vi "BusTapeFiducialAnalysis.vi"() -> ()   [LabVIEW 2016]
uses:
  <vilib>/vision/Image Controls.llb/IMAQ Image.ctl
  <vilib>/vision/Measure.llb/Edge Options.ctl
  <vilib>/vision/Measure.llb/Edge Polarity.ctl
  <vilib>/Analysis/6fits.llb/Curve Fitting Criteria.ctl
  <vilib>/Utility/file.llb/Write Delimited Spreadsheet (DBL).vi
  <vilib>/vision/NI_Vision_Development_Module.lvlib
  <vilib>/Analysis/NI_AALPro.lvlib
  <vilib>/Analysis/NI_AALBase.lvlib
panel:
  out "Std Dev":dbl
  out "Mean":dbl
  out "Fit Deviation":T1(graph)
  out "Fiducial spacing (mm)\n(bottom)":dbl[](array[numeric])
  out "Fiducial spacing (mm)\n(top)":dbl[](array[numeric])
  out "Deviation from Fit (um)":dbl[](array[numeric])
  out "Mean Location Error (um)":dbl[][](array[numeric])
  out "Mean Location (mm)":dbl[][](array[numeric])
  out "Fiducial 14 Y":cluster{i32[], dbl[]}(graph)
  out "Fiducial 14 X":cluster{i32[], dbl[]}(graph)
  out "Fiducial 13 Y":cluster{i32[], dbl[]}(graph)
  out "Fiducial 13 X":cluster{i32[], dbl[]}(graph)
  out "Fiducial 12 Y":cluster{i32[], dbl[]}(graph)
  out "Fiducial 12 X":cluster{i32[], dbl[]}(graph)
  out "Fiducial 11 Y":cluster{i32[], dbl[]}(graph)
  out "Fiducial 11 X":cluster{i32[], dbl[]}(graph)
  out "Fiducial 10 Y":cluster{i32[], dbl[]}(graph)
  out "Fiducial 10 X":cluster{i32[], dbl[]}(graph)
  out "Fiducial 9 Y":cluster{i32[], dbl[]}(graph)
  out "Fiducial 9 X":cluster{i32[], dbl[]}(graph)
  out "Fiducial 8 Y":cluster{i32[], dbl[]}(graph)
  out "Fiducial 8 X":cluster{i32[], dbl[]}(graph)
  out "Fiducial 7 Y":cluster{i32[], dbl[]}(graph)
  out "Fiducial 7 X":cluster{i32[], dbl[]}(graph)
  out "Fiducial 6 Y":cluster{i32[], dbl[]}(graph)
  out "Fiducial 6 X":cluster{i32[], dbl[]}(graph)
  out "Fiducial 5 Y":cluster{i32[], dbl[]}(graph)
  out "Fiducial 5 X":cluster{i32[], dbl[]}(graph)
  out "Fiducial 4 Y":cluster{i32[], dbl[]}(graph)
  out "Fiducial 4 X":cluster{i32[], dbl[]}(graph)
  out "Fiducial 3 Y":cluster{i32[], dbl[]}(graph)
  out "Fiducial 3 X":cluster{i32[], dbl[]}(graph)
  out "Fiducial 2 Y":cluster{i32[], dbl[]}(graph)
  out "Fiducial 2 X":cluster{i32[], dbl[]}(graph)
  out "Fiducial 1 Y":cluster{i32[], dbl[]}(graph)
  out "Fiducial 1 X":cluster{i32[], dbl[]}(graph)
  out "Fiducial Loc":dbl[][](array[numeric])
  out "Drift 2":cluster{dbl[], dbl[]}(graph)
  out "Radius [um] 2":dbl[](array[numeric])
  out "Derivative: Normalized Intensity vs Radius":T2(graph)
  out "Normalized Intensity vs Radius":cluster{dbl[], dbl[]}(graph)
  in  "nBins":dbl=300.0
  in  "Min":dbl
  in  "Max":dbl=300.0
  out "Npixel@Intensity Histogram":T1(graph)
  out "Npixel@phi Histogram":T1(graph)
  out "Npixel@R Histogram":T1(graph)
  out "Bottom Intercept\n(mm)":dbl
  out "Bottom Slope\n(um/mm)":dbl
  out "Top Intercept\n(mm)":dbl
  out "Top Slope\n(um/mm)":dbl
  out "Pixel to Micron Conversion":T1(graph)
  out "Bottom errors (um)":dbl[](array[numeric])
  out "Top errors (um)":dbl[](array[numeric])
  out "Scaling [um/px]":dbl[](array[numeric])
  out "Bottom":cluster{"Bottom":dbl[], "Bottom":dbl[]}[](graph)
  out "Bottom \nResiduals (um)":dbl[](array[numeric])
  out "Radius [um]":dbl[](array[numeric])
  out "Top \nResiduals (um)":dbl[](array[numeric])
  out "Top":cluster{"Top":dbl[], "Top":dbl[]}[](graph)
  in  "method":T3 items=["Least Square", "Least Absolute Residual", "Bisquare"]
  out "Bottom":dbl[][](array[numeric])
  out "Top":dbl[][](array[numeric])
  out "Coordinate array for image capture":dbl[][](array[numeric])
  out "Processing Image #":i32
  out "Selected subarray":T4(plugin-control)
  out "Fitted Circle":T5 {"Average SNR (dB)" format="%.2f"; "Average Strength" format="%.2f"; "Roundness (Real-World)" format="%.2f"; "Radius (Real-World)" format="%.2f"; "Center (Real-World)"."Y" format="%.2f"; "Center (Real-World)"."X" format="%.2f"; "Radius (Pixels)" format="%.2f"; "Center (Pixels)"."Y" format="%.2f"; "Center (Pixels)"."X" format="%.2f"}
  in  "Circle ROI Descriptor":T6={"Global Rectangle"=[675, 567, 1751, 1642], "Contours"=[{"ID"=enum."External", "Type"=7, "Coordinates"=[1212, 1104, 190, 250, 0, 0]}]} {"Contours"."Type" items=["No Selection", "Point", "Line", "Rectangle", "Oval", "Polygon", "Freehand Region", "Annulus", "Unused2", "Unused3", "Broken Line", "Freehand Line", "Rotated Rectangle"]}
  in  "Circle Fit Options":T7={"Process"=enum."Get Best Edge", "Step Size"=3.0, "Max Pixel Radius"=3}
  in  "Circle Finding Options":T10={"Search  Direction"=1, "Edge Options"={"Edge Polarity"=2, "Kernel Size"=3, "Width"=3, "Minimum Edge Strength"=10.0, "Interpolation Type"=enum."Bilinear Fixed", "Data Processing Method"=enum."Median"}, "Show Search Area"=TRUE, "Show Search Lines"=TRUE, "Show Edges Found"=TRUE, "Show Result"=TRUE, "Search Area Color"=65280, "Search Lines Color"=255, "Edge Locations Color"=16776960, "Result Color"=65511, "Overlay Group Name"=""} {"Search  Direction" items=["Outside to Inside", "Inside to Outside"]; "Edge Options"."Edge Polarity" items=["All Edges", "Rising Edges", "Falling Edges"]; "Edge Options"."Minimum Edge Strength" format="%.2f"; "Edge Options"."Width" step=2; "Edge Options"."Kernel Size" step=2}
  in  "Pattern Match Settings":T11={"Algorithm"=2, "Number of Matches Requested"=1, "Minimum Match Score"=800.0, "SubPixel Accuracy"=TRUE, "Rotation Angle Ranges"=[], "Show Search Area"=FALSE, "Show Result"=TRUE} {"Rotation Angle Ranges"."End" format="%.1f"; "Rotation Angle Ranges"."Start" format="%.1f"; "Minimum Match Score" min=0 max=1000 format="%.2f"; "Number of Matches Requested" min=1; "Algorithm" items=["All", "Low Discrepancy Sampling", "Grayscale Value Pyramid", "Gradients Pyramid"]}
  out "Template Image":T4
  in  "Coordinate file for image capture":path=path "D:/Git/StaveAssembly/XYZstage+Camera_CollectedImages/2017-03-15/BrendonsFidMarks_dots_2017-03-15-captured.csv"
  out "Review":bool
  out "Search running?":bool
  in  "Stop and delete":bool
  out "Images Array":T4[](array[plugin-control])=["image_442_-22_00"]
  in  "error in":errorcluster
  out "error out":errorcluster
  out "Filenames Array":string[](array[string])=["image_442_-22_110.png", "image_442_-22_137.png", "image_442_-22_192.png", "image_442_-22_222.png", "image_442_-22_26.png", "image_442_-22_56.png"]
  in  "Naming Convention":string="image_*_*_*_*.png"
  in  "Images Directory":path=path "D:/Git/StaveAssembly/XYZstage+Camera_CollectedImages/2017-03-15/images"
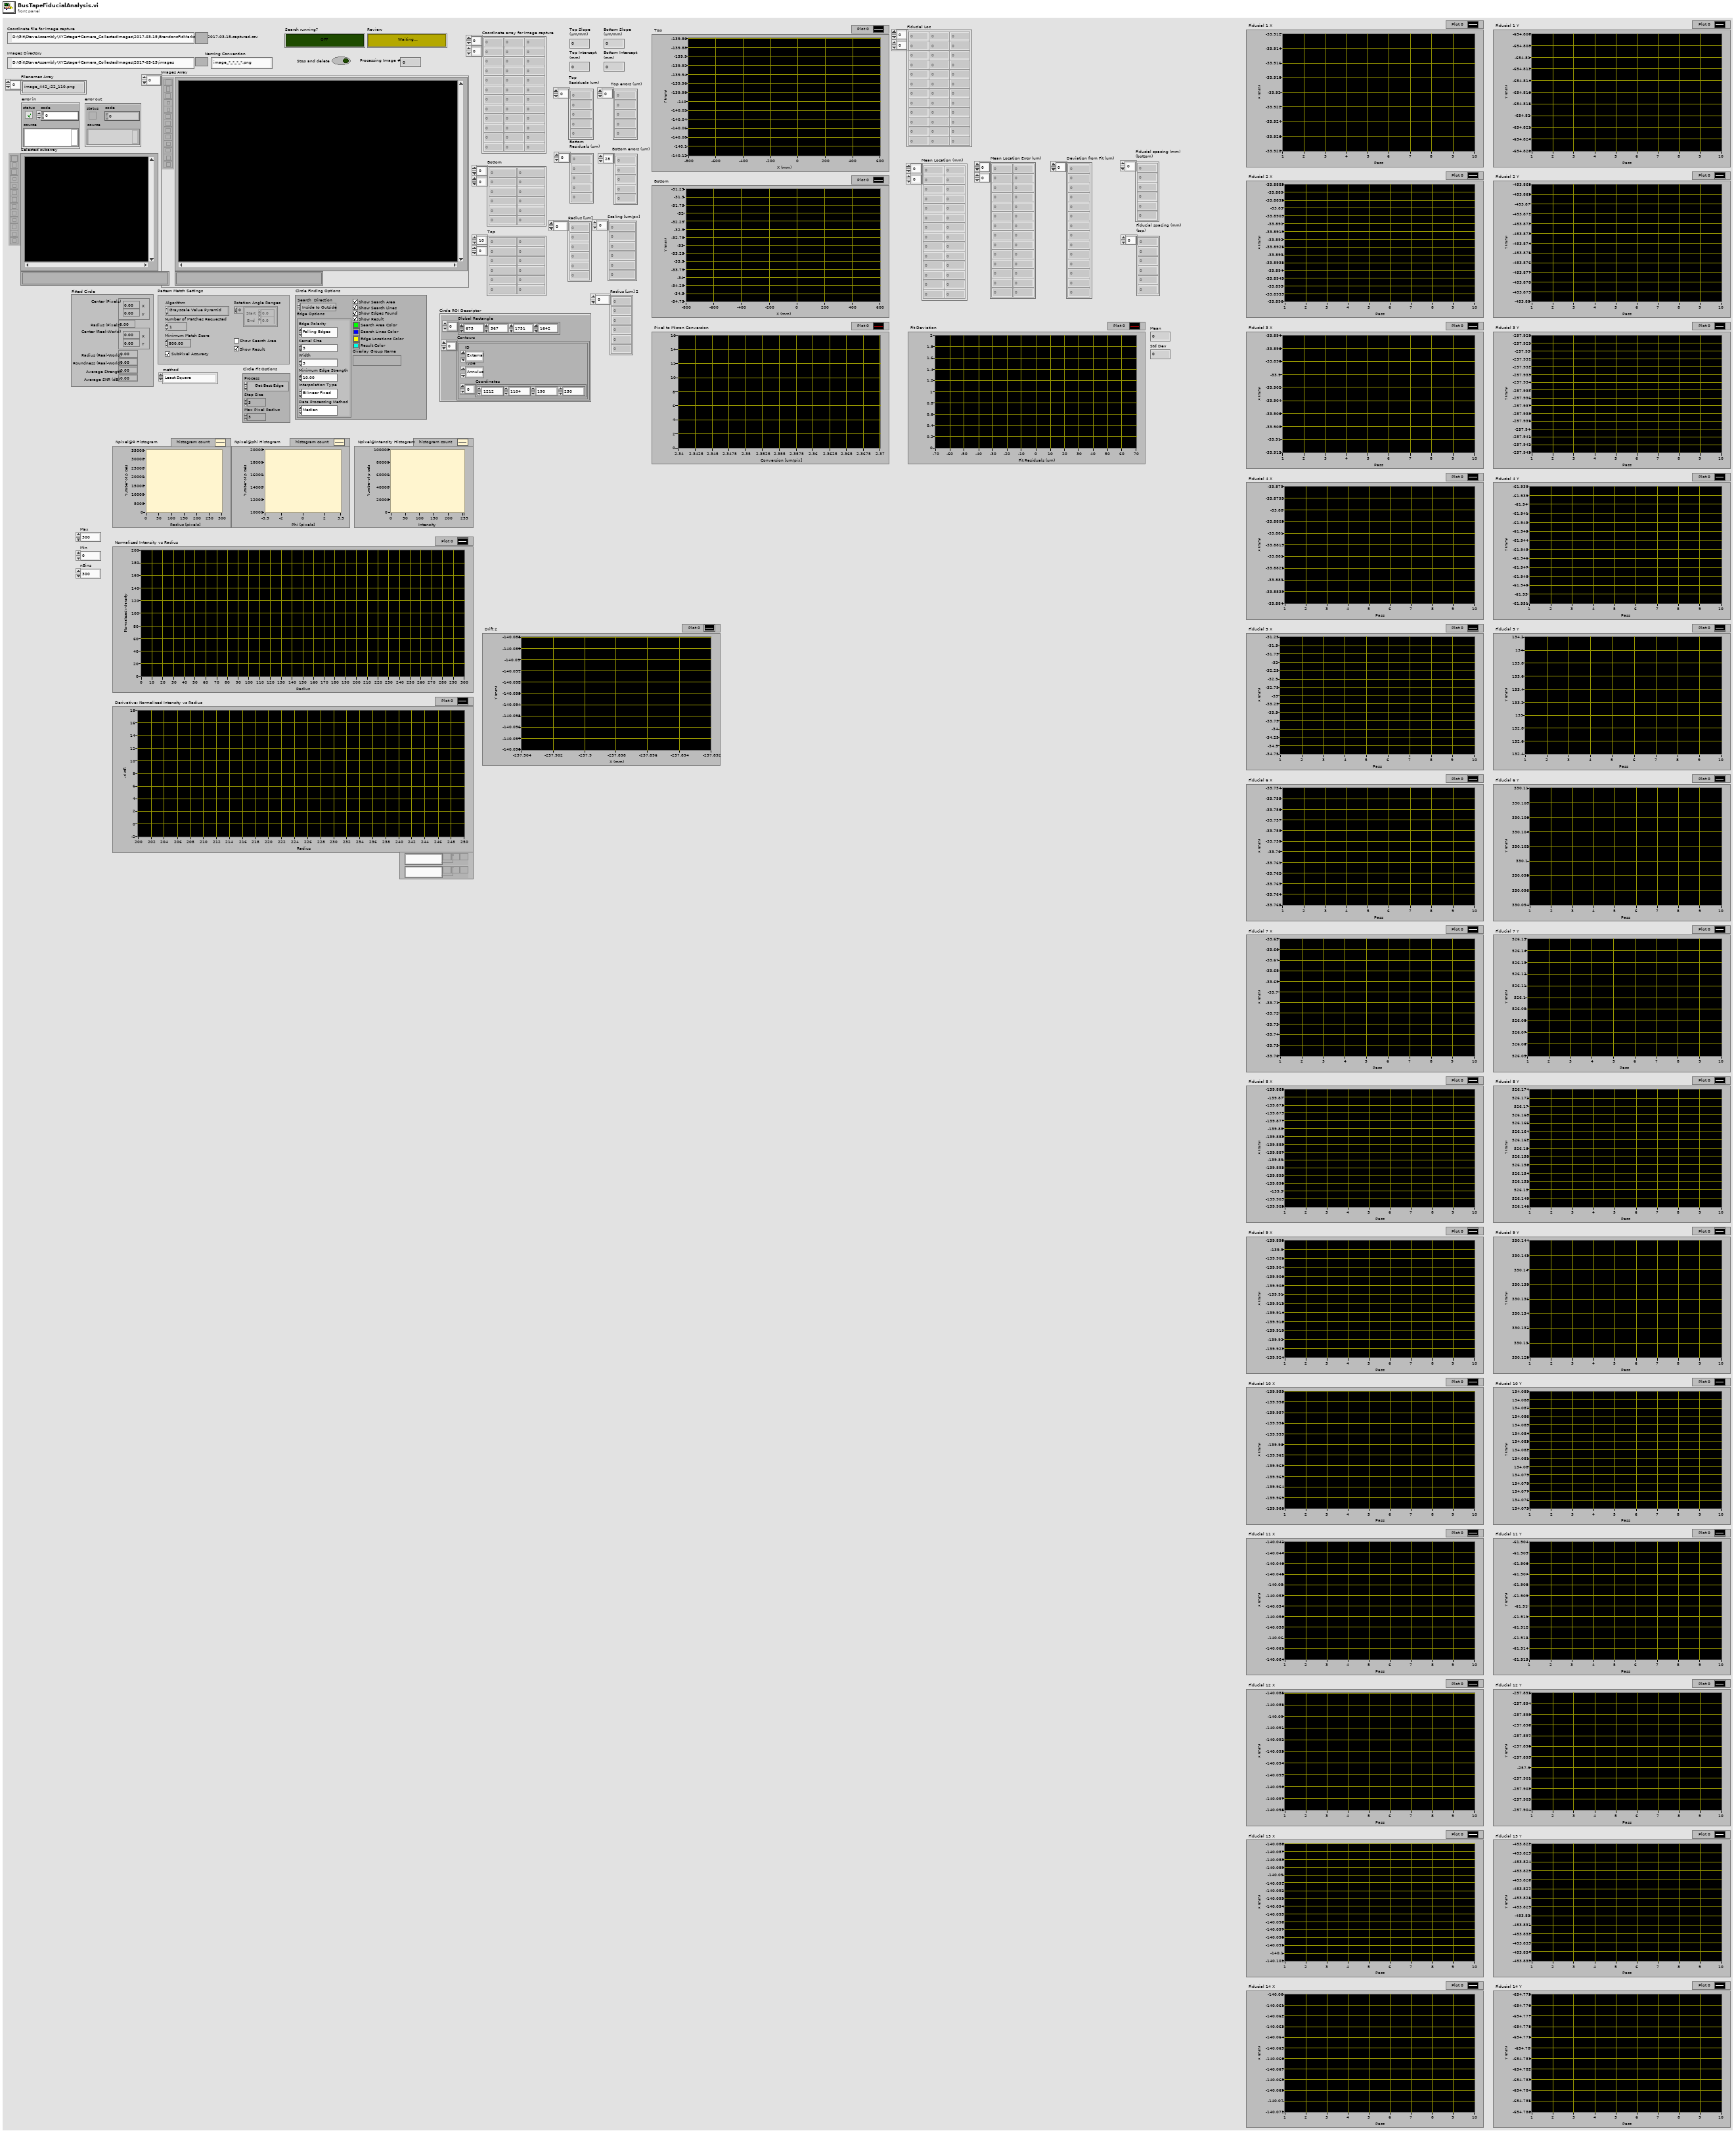
[diagram p1: front panel]
types:
  T1 = cluster{"X Values":dbl[], "Histogram: h(x)":i32[]}
  T2 = cluster{"Radius bins":dbl[], "Best Gaussian Fit":dbl[]}[]
  T3 = typedef "NI_AALPro.lvlib/Curve Fitting Criteria.ctl" = u16
  T4 = typedef "IMAQ Image.ctl" = refnum<image>
  T5 = cluster{"Center (Pixels)":cluster{"X":sgl, "Y":sgl}, "Radius (Pixels)":dbl, "Center (Real-World)":cluster{"X":sgl, "Y":sgl}, "Radius (Real-World)":dbl, "Roundness (Real-World)":dbl, "Average Strength":dbl, "Average SNR (dB)":dbl}
  T6 = cluster{"Global Rectangle":i32[], "Contours":cluster{"ID":enum32{"External", "Internal"}, "Type":u32, "Coordinates":i32[]}[]}
  T7 = cluster{"Process":enum16{"Get First Edge", "Get First + Last Edge", "Get All Edges", "Get Best Edge"}, "Step Size":dbl, "Max Pixel Radius":i32}
  T8 = typedef "Edge Options.ctl" = cluster{"Edge Polarity":T9, "Kernel Size":u32, "Width":u32, "Minimum Edge Strength":sgl, "Interpolation Type":enum32{"Zero Order", "Bilinear", "Quadratic", "Cubic", "Bilinear Fixed"}, "Data Processing Method":enum32{"Average", "Median"}}
  T9 = typedef "Edge Polarity.ctl" = u32
  T10 = cluster{"Search  Direction":u32, "Edge Options":T8, "Show Search Area":bool, "Show Search Lines":bool, "Show Edges Found":bool, "Show Result":bool, "Search Area Color":u32, "Search Lines Color":u32, "Edge Locations Color":u32, "Result Color":u32, "Overlay Group Name":string}
  T11 = cluster{"Algorithm":i32, "Number of Matches Requested":i32, "Minimum Match Score":sgl, "SubPixel Accuracy":bool, "Rotation Angle Ranges":cluster{"Start":sgl, "End":sgl}[], "Show Search Area":bool, "Show Result":bool}
  T12 = enum16{"Get First Edge", "Get First + Last Edge", "Get All Edges", "Get Best Edge"}
  T13 = typedef "Search Line.ctl" = cluster{"Start Point":cluster{"X":sgl, "Y":sgl}, "End Point":cluster{"X":sgl, "Y":sgl}, "Edge Info":T14[], "Edge Map":dbl[], "Calibration Valid":bool}
  T14 = typedef "Edge New.ctl" = cluster{"Location (Pixel)":cluster{"X":sgl, "Y":sgl}, "Location (Real-World)":cluster{"X":sgl, "Y":sgl}, "Distance (Pixel)":dbl, "Distance (Real-World)":dbl, "Strength":dbl, "Noise":dbl, "Rising?":bool}
  T15 = cluster{"Position":cluster{"x":sgl, "y":sgl}, "Angle":sgl, "Scale":sgl, "Score":sgl, "Bounding Box":cluster{"x":sgl, "y":sgl}[]}[]
  T16 = cluster{"Global Rectangle":i32[], cluster{"ID":enum32{"External", "Internal"}, "Type":u32, "Coordinates":i32[]}[]}
  T17 = cluster{"initial amplitude":dbl, "initial center":dbl, "initial standard deviation":dbl, "offset":dbl}
  T18 = cluster{"Radius bins":dbl[], "Normalized Intensity":dbl[]}
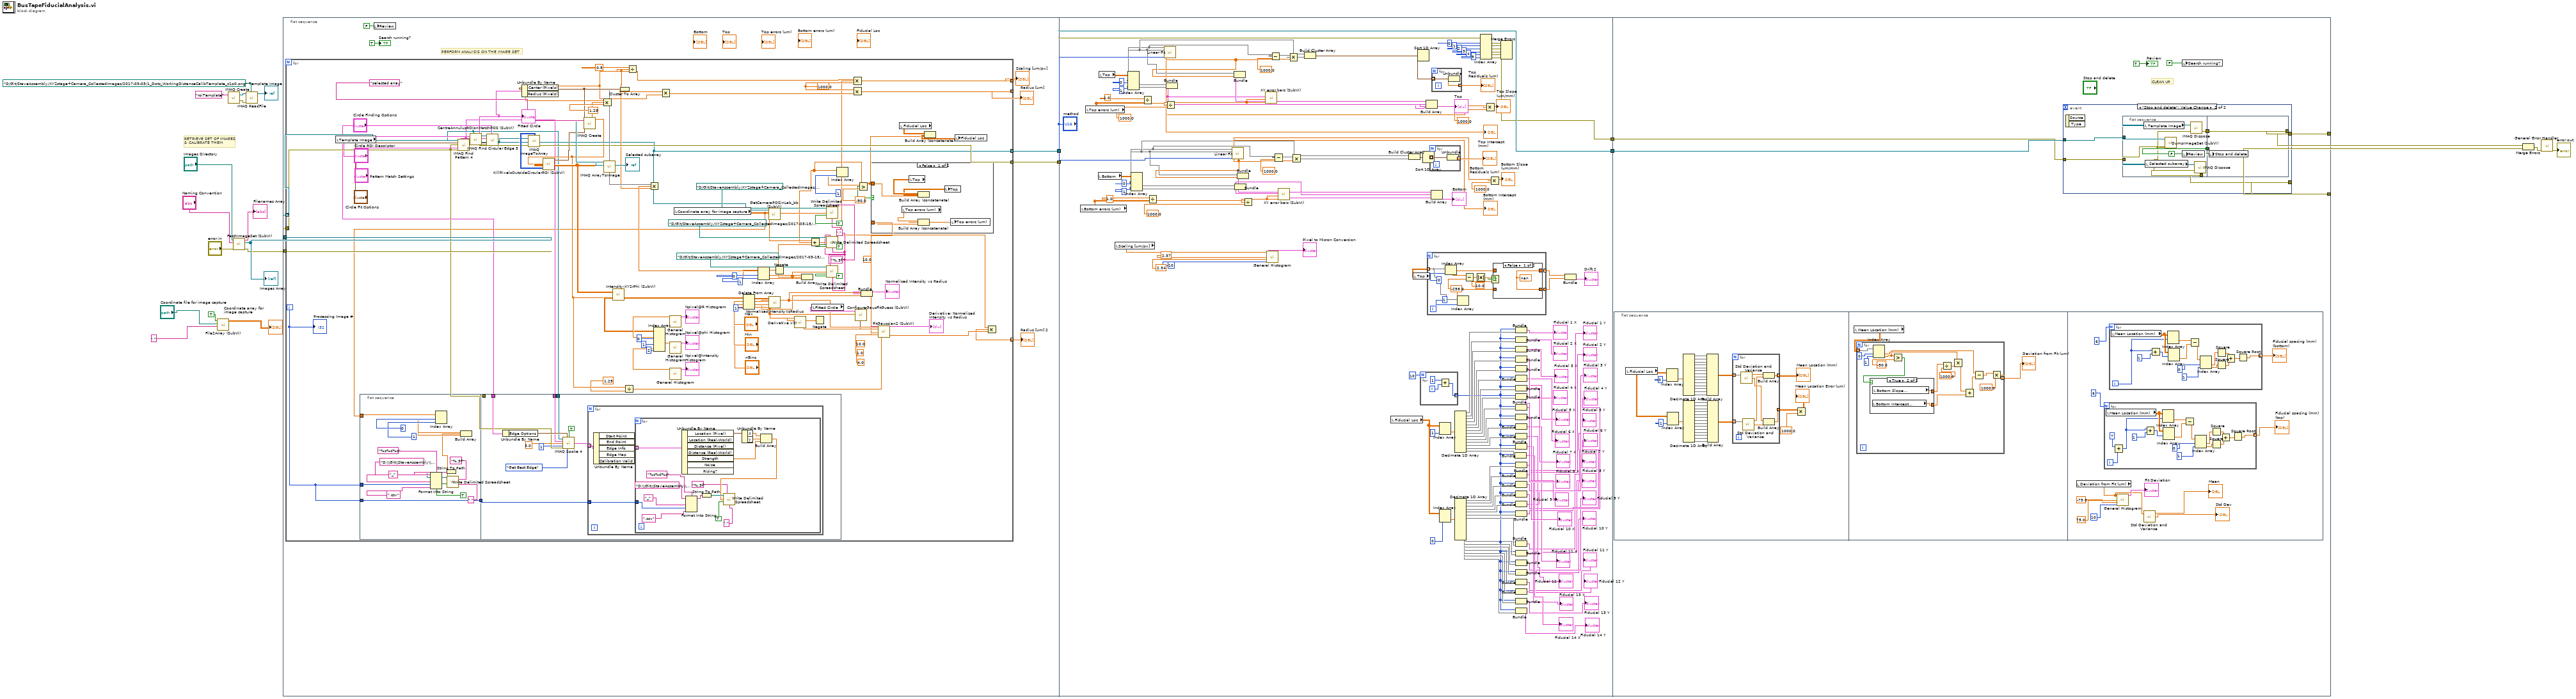
[diagram p0: block diagram]
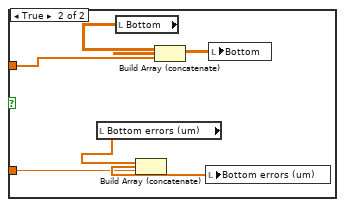
[diagram p2: hidden frame]
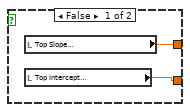
[diagram p4: hidden frame]
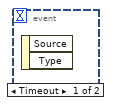
[diagram p5: hidden frame]
diagram:
  # "RETRIEVE SET OF IMAGES\n& CALIBRATE THEM"
  n1 = call "File2Array (SubVI).vi"("File delimiter"=",", "Source array file"="Coordinate file for image capture", "Load array from file?"=TRUE) -> ("Loaded array"=→"Coordinate array for image capture":dbl[][])  [unwired: 7 in, 1 out]
  n2 = call "IMAQ Create"("Image Name"="roiTemplate") -> ("New Image"=w2:T4, "error out"=w14:errorcluster)  [unwired: 4 in]
  n3 = call "FetchImageSet (SubVI).vi"("error in (no error)"="error in", "Naming Convention"="Naming Convention", "Images Directory"="Images Directory") -> ("error out"=w12:errorcluster, "Image Array"=w16:T4[], "Filenames Array"=→"Filenames Array":string[])  [unwired: 6 in]
  "Images Array" <- w16
  n4 = call "IMAQ ReadFile"("File Path"=path "D:/Git/StaveAssembly/XYZstage+Camera_CollectedImages/2017-03-03/1_Dots_WorkingDistanceCalibTemplate_z1p0.png" ("Template File Path"), "error in (no error)"=w14, "Image"=w2) -> ("Image Out"=→"Template Image":T4)  [unwired: 4 in, 4 out]
  n5 = flat-sequence {
    tunnel: w16 -> [w30]
    tunnel: w12 -> [w29]
    tunnel: [w28] -> w5
    tunnel: [w27] -> w4
    tunnel: [w314] -> w11
    tunnel: w5 -> [w314]
    tunnel: w4 -> [w312]
    tunnel: [w313] -> w3
    tunnel: [w340] -> w18
    tunnel: w11 -> [w339]
    tunnel: [w338] -> w10
    tunnel: w3 -> [w337]
    frame #0 {
      # "PERFORM ANALYSIS ON THE IMAGE SET"
      n6 = for {
        tunnel: w30 -> [w119] mode=indexing
        tunnel: w29 -> [w117]
        tunnel: [w78] -> w28 mode=indexing
        tunnel: [w87] -> w27 mode=indexing
        tunnel: [w44] -> w26 mode=indexing
        tunnel: [w81] -> w25 mode=indexing
        tunnel: [w43] -> w24 mode=indexing
        i -> [w36]
        (unwired) 10.0
        w82 = 1000.0
        w92 = "," ("File delimiter")
        w95 = "%.3f"
        n7 = local read "Template Image"() -> (w80:T4)
        n8 = flat-sequence {
          tunnel: w36 -> [w136]
          tunnel: [w136] -> w38
          tunnel: w37 -> [w135]
          tunnel: w36 -> [w125]
          tunnel: "Circle Finding Options" -> [w147]
          tunnel: w41 -> [w144]
          tunnel: w40 -> [w143]
          tunnel: w39 -> [w142]
          tunnel: w38 -> [w137]
          frame #0 {
            n9 = Format Into String(format string="%s%d%s", initial string="D:\\Git\\StaveAssembly\\XYZstage+Camera_CollectedImages\\2017-03-15\\out\\circleEdges", "_", w125, ".csv") -> (resulting string=w131:string)  [unwired: 1 in, 1 out]
            n10 = Index Array(array=w135, index #1=0, index #2=1) -> (element #1=w123:dbl, element #2=w122:dbl)
            n11 = String To Path(string=w131) -> (path=w130:path)
            n12 = Build Array(w123, w122) -> (w121:dbl[])
            n13 = call-poly <vilib>:"Write Delimited Spreadsheet.vi"("file path (dialog if empty)"=w130, "format (%.3f)"="%.3f", "1D data"=w121, "append to file? (new file:F)"=TRUE, "delimiter (\\t)"="," ("File delimiter")) -> ()  [unwired: 9 in, 2 out]
          }
          frame #1 {
            n14 = Unbundle By Name(w147) -> ("Edge Options"=w146:T8)
            n15 = call "IMAQ Spoke 4"("Image"=w144, "Edge Options"=w146, "Optimized Mode"=TRUE, "ROI Descriptor"=w143, "Step Size"=3.0, "Scan Direction"=1, "error in (no error)"=w142, "Process"=T12."Get Best Edge") -> ("Search Lines"=w138:T13[])  [unwired: 4 in, 3 out]
            n16 = for {
              tunnel: w138 -> [w150] mode=indexing
              tunnel: w137 -> [w148]
              n17 = Unbundle By Name(w150) -> ("Edge Info"=w149:T14[])  [unwired: 4 out]
              n18 = for {
                tunnel: w149 -> [w163] mode=indexing
                tunnel: w148 -> [w162]
                n19 = Unbundle By Name(w163) -> ("Location (Pixel)"=w160:cluster{"X":sgl, "Y":sgl}, "Strength"=w157:dbl)  [unwired: 5 out]
                n20 = Format Into String(format string="%s%d%s", initial string="D:\\Git\\StaveAssembly\\XYZstage+Camera_CollectedImages\\2017-03-15\\out\\circleEdges", "_", w162, ".csv") -> (resulting string=w165:string)  [unwired: 1 in, 1 out]
                n21 = String To Path(string=w165) -> (path=w164:path)
                n22 = Unbundle By Name(w160) -> ("X"=w159:sgl, "Y"=w158:sgl)
                n23 = Build Array(w159, w158, w157) -> (w156:dbl[])
                n24 = call-poly <vilib>:"Write Delimited Spreadsheet.vi"("file path (dialog if empty)"=w164, "format (%.3f)"="%.3f", "1D data"=w156, "append to file? (new file:F)"=TRUE, "delimiter (\\t)"="," ("File delimiter")) -> ()  [unwired: 9 in, 2 out]
              }
            }
          }
        }
        n25 = call "IMAQ Find Pattern 4"("Image"=w119, "Template"=w80, "error in"=w117, "Settings"="Pattern Match Settings") -> ("Image Out"=w41:T4, "Matches (pixel)"=w114:T15, "error out"=w39:errorcluster)  [unwired: 5 in, 4 out]
        n26 = call "CentreAnnulusROIonMatchPOS (SubVI).vi"("Matches (pixel)"=w114, "Annulus ROI Descriptor"="Circle ROI Descriptor") -> ("Annulus ROI Descriptor centred on match position"=w40:T16)
        n27 = call "IMAQ Find Circular Edge 3"("Circle Fit Options"="Circle Fit Options", "Options"="Circle Finding Options", "error in (no error)"=w39, "ROI Descriptor"=w40, "Image"=w41) -> ("error out"=w87:errorcluster, "Fitted Circle"=w108:T5, "Image Out"=w78:T4)  [unwired: 2 in, 2 out]
        "Fitted Circle" <- w108
        n28 = Unbundle By Name(w108) -> ("Center (Pixels)"=w107:cluster{"X":sgl, "Y":sgl}, "Radius (Pixels)"=w85:dbl)
        n29 = call "IMAQ ImageToArray"("error in (no error)"=w87, "Image"=w78) -> ("Image Pixels (U8)"=w112:u8[][])  [unwired: 2 in, 4 out]
        n30 = call "IMAQ Create"("Image Name"="selected array") -> ("New Image"=w110:T4)  [unwired: 4 in, 1 out]
        n31 = Multiply(x=w85, y=1.25) -> (x*y=w48:dbl)
        n32 = call "KillPixelsOutsideCircularROI (SubVI).vi"("XY Array"=w112, "Radius*ScaleFactor"=w48, "Center (Pixels)"=w107) -> ("subarray"=w76:dbl[][])
        n33 = call "IMAQ ArrayToImage"("Image Pixels (U8)"=w76, "Image"=w110) -> ("Image Out"=→"Selected subarray":T4)  [unwired: 8 in, 1 out]
        n34 = call "Intensity-XY2rPhi (SubVI).vi"("Radius*Scale Factor"=w48, "XY Array"=w76) -> ("2D Array: r, phi, intensity"=w66:dbl[][])  [unwired: 1 out]
        n35 = Cluster To Array(cluster=w107) -> (array=w106:sgl[])
        n36 = Divide(x=w48, y=1.25) -> (x/y=w47:dbl)
        n37 = Divide(x=0.5, y=w85) -> (x/y=w84:dbl)
        n38 = Multiply(x=w106, y=w84) -> (x*y=w101:dbl[])
        n39 = Index Array(array=w66, index (col) #1=0 ("disabled index (col)"), index (col) #2=1 ("index (col)"), index (col) #3=2 ("index (col)")) -> (element #1=w68:dbl[], element #2=w69:dbl[], element #3=w67:dbl[])  [unwired: 3 in]
        n40 = Multiply(x=w84, y=w85) -> (x*y=w83:dbl)
        n41 = call <vilib>:"General Histogram.vi"("X"=w68) -> ("Histogram Graph"=→"Npixel@R Histogram":T1)  [unwired: 10 in, 4 out]
        n42 = call <vilib>:"General Histogram.vi"("X"=w69) -> ("Histogram Graph"=→"Npixel@phi Histogram":T1)  [unwired: 10 in, 4 out]
        n43 = call <vilib>:"General Histogram.vi"("X"=w67) -> ("Histogram Graph"=→"Npixel@Intensity Histogram":T1)  [unwired: 10 in, 4 out]
        n44 = local read "Coordinate array for image capture"() -> (w79:dbl[][])
        n45 = Delete From Array(array=w66, index (col)=1 ("disabled index (col)")) -> (array with subset deleted=w64:dbl[][])  [unwired: 2 in, 1 out]
        n46 = Index Array(array=w101, index #1=0, index #2=1) -> (element #1=w97:dbl, element #2=w98:dbl)
        n47 = call "GetCameraPOSinLab_bb (SubVI).vi"("Loaded array"=w79, "Refnum in"=w78) -> ("Image coordinates in lab frame"=w37:dbl[])  [unwired: 7 in, 2 out]
        n48 = call "NormalizedIntensityVsRadius.vi"("nBins"="nBins", "Min"="Min", "Max"="Max", "Input Array (r,I)"=w64) -> ("Normalized Intensity"=w53:dbl[], "Radius bins"=w57:dbl[])  [unwired: 5 in, 1 out]
        n49 = Negate(x=w98) -> (-x=w96:dbl)
        n50 = call <vilib>:"Derivative x(t).vi"("X"=w53) -> ("dX/dt"=w60:dbl[])  [unwired: 9 in, 1 out]
        n51 = Build Array(w96, w97) -> (w77:dbl[])
        n52 = Add(x=w37, y=w77) -> (x+y=w33:dbl[])
        n53 = local read "Fitted Circle"() -> (w59:T5)
        n54 = Negate(x=w60) -> (-x=w58:dbl[])
        n55 = call-poly <vilib>:"Write Delimited Spreadsheet.vi"("file path (dialog if empty)"=path "D:/Git/StaveAssembly/XYZstage+Camera_CollectedImages/2017-03-15/imageLocation.csv", "format (%.3f)"=w95, "1D data"=w37, "append to file? (new file:F)"=TRUE, "delimiter (\\t)"=w92) -> ()  [unwired: 9 in, 2 out]
        n56 = call-poly <vilib>:"Write Delimited Spreadsheet.vi"("file path (dialog if empty)"=path "D:/Git/StaveAssembly/XYZstage+Camera_CollectedImages/2017-03-15/labFrame.csv", "format (%.3f)"=w95, "1D data"=w33, "append to file? (new file:F)"=TRUE, "delimiter (\\t)"=w92) -> ()  [unwired: 9 in, 2 out]
        n57 = call-poly <vilib>:"Write Delimited Spreadsheet.vi"("file path (dialog if empty)"=path "D:/Git/StaveAssembly/XYZstage+Camera_CollectedImages/2017-03-15/imageFrame.csv", "format (%.3f)"=w95, "1D data"=w77, "append to file? (new file:F)"=TRUE, "delimiter (\\t)"=w92) -> ()  [unwired: 9 in, 2 out]
        n58 = Index Array(array=w33, index=1) -> (element=w90:dbl)
        n59 = Multiply(x=w84, y=w82) -> (x*y=w44:dbl)
        n60 = Multiply(x=w82, y=w83) -> (x*y=w81:dbl)
        n61 = call "ConfigureGausFitGuess (SubVI).vi"("Array"=w53, "Fitted Circle"=w59) -> ("initial guess out"=w56:T17)  [unwired: 9 in]
        n62 = Greater?(x=w90, y=-90.0) -> (0:w88:bool)
        n63 = Bundle("Radius bins"=w57, "Normalized Intensity"=w53) -> (→"Normalized Intensity vs Radius":T18)  [unwired: 1 in]
        n64 = call "FitGaussian2 (SubVI).vi"("x values"=w57, "y values"=w58, "Estimated mean"=w47, "initial guess"=w56, "Estimated width"=10.0, "Nsigma Low"=1.0, "Nsigma High"=4.0) -> ("Plot with Gaussian fit"=→"Derivative: Normalized Intensity vs Radius":T2, "center"=w45:dbl, "standard deviation"=w46:dbl)  [unwired: 7 in, 3 out]
        n65 = case shown="False" w88 {
          tunnel: w33 -> [w167 w177]
          tunnel: w46 -> [w168 w173]
          frame False {
            n66 = local read "Top errors (um)"() -> (w170:dbl[])
            n67 = local read "Top"() -> (w172:dbl[][])
            n68 = Build Array (concatenate)(w170, w168) -> (w169:dbl[])
            n69 = Build Array (concatenate)(w172, w167) -> (w171:dbl[][])
            n70 = local write "Top"(w171) -> ()
            n71 = local write "Top errors (um)"(w169) -> ()
          }
          frame True {
            n72 = local read "Bottom errors (um)"() -> (w175:dbl[])
            n73 = local read "Bottom"() -> (w178:dbl[][])
            n74 = Build Array (concatenate)(w175, w173) -> (w174:dbl[])
            n75 = Build Array (concatenate)(w178, w177) -> (w176:dbl[][])
            n76 = local write "Bottom errors (um)"(w174) -> ()
            n77 = local write "Bottom"(w176) -> ()
          }
        }
        n78 = local read "Fiducial Loc"() -> (w34:dbl[][])
        n79 = Build Array (concatenate)(w34, w33) -> (w35:dbl[][])
        n80 = local write "Fiducial Loc"(w35) -> ()
        n81 = Multiply(x=w44, y=w45) -> (x*y=w43:dbl)
        "Processing Image #" <- w36
      }
      "Scaling [um/px]" <- w26
      "Radius [um]" <- w25
      "Radius [um] 2" <- w24
      n82 = local write "Review"(FALSE ("Review")) -> ()
      "Search running?" <- TRUE ("Search running?")
    }
    frame #1 {
      n83 = local read "Bottom errors (um)"() -> (w262:dbl[])
      n84 = local read "Top errors (um)"() -> (w263:dbl[])
      n85 = local read "Bottom"() -> (w293:dbl[][])
      n86 = local read "Top"() -> (w299:dbl[][])
      n87 = local read "Scaling [um/px]"() -> (w258:dbl[])
      n88 = Index Array(array=w299, index (col) #1=0, index (col) #2=1) -> (element #1=w278:dbl[], element #2=w272:dbl[])  [unwired: 2 in]
      n89 = Index Array(array=w293, index (col) #1=0, index (col) #2=1) -> (element #1=w284:dbl[], element #2=w274:dbl[])  [unwired: 2 in]
      n90 = Divide(x=1.0, y=w263) -> ()  [unwired: 1 out]
      n91 = Divide(x=1.0, y=w262) -> ()  [unwired: 1 out]
      n92 = call <vilib>:"Linear Fit.vi"("Y"=w272, "X"=w278, "method"="method") -> ("Best Linear Fit"=w273:dbl[], "slope"=w247:dbl, "intercept"=→"Top Intercept\n(mm)":dbl)  [unwired: 8 in, 2 out]
      n93 = Divide(x=w263, y=1000.0) -> (x/y=w265:dbl[])
      n94 = Bundle("Top"=w278, "Top"=w272) -> (w266:cluster{"Top":dbl[], "Top":dbl[]})  [unwired: 1 in]
      n95 = call <vilib>:"Linear Fit.vi"("Y"=w274, "X"=w284, "method"="method") -> ("Best Linear Fit"=w275:dbl[], "slope"=w250:dbl, "intercept"=→"Bottom Intercept\n(mm)":dbl)  [unwired: 8 in, 2 out]
      n96 = Bundle("Top"=w278, "Best Linear Fit"=w273) -> (w296:cluster{"Top":dbl[], "Best Linear Fit":dbl[]})  [unwired: 1 in]
      n97 = Bundle("Bottom"=w284, "Bottom"=w274) -> (w271:cluster{"Bottom":dbl[], "Bottom":dbl[]})  [unwired: 1 in]
      n98 = Bundle("Bottom"=w284, "Best Linear Fit"=w275) -> (w290:cluster{"Bottom":dbl[], "Best Linear Fit":dbl[]})  [unwired: 1 in]
      n99 = Divide(x=w262, y=1000.0) -> (x/y=w269:dbl[])
      n100 = call "XY error bars (SubVI).vi"("XY plot"=w266, "Xerror"=w265, "Yerror"=w265) -> ("X+Y error bars"=w260:cluster{dbl[], dbl[]})  [unwired: 5 in, 2 out]
      n101 = call <vilib>:"General Histogram.vi"("X"=w258, "max"=2.37, "min"=2.34, "# bins"=10) -> ("Histogram Graph"=→"Pixel to Micron Conversion":T1)  [unwired: 7 in, 4 out]
      n102 = Subtract(x=w272, y=w273) -> (x-y=w295:dbl[])
      n103 = Subtract(x=w274, y=w275) -> (x-y=w289:dbl[])
      n104 = call "XY error bars (SubVI).vi"("XY plot"=w271, "Xerror"=w269, "Yerror"=w269) -> ("X+Y error bars"=w259:cluster{dbl[], dbl[]})  [unwired: 5 in, 2 out]
      n105 = Multiply(x=w295, y=1000.0) -> (x*y=w280:dbl[])
      n106 = Multiply(x=w289, y=1000.0) -> (x*y=w285:dbl[])
      n107 = Build Cluster Array(w278, w280) -> (w279:cluster{"Numeric":dbl, dbl}[])
      n108 = local read "Fiducial Loc"() -> (w207:dbl[][])
      n109 = Build Cluster Array(w284, w285) -> (w283:cluster{"Numeric":dbl, dbl}[])
      n110 = local read "Top"() -> (w245:dbl[][])
      n111 = Sort 1D Array(array=w279) -> (sorted array=w277:cluster{"Numeric":dbl, dbl}[])
      n112 = for {
        N: 10 -> [_]
        tunnel: [w316] -> w208 mode=indexing
        i -> [w317]
        n113 = Add(x=1, y=w317) -> (x+y=w316:i32)
      }
      n114 = Sort 1D Array(array=w283) -> (sorted array=w282:cluster{"Numeric":dbl, dbl}[])
      n115 = Build Array(w296, w266, w260) -> (→"Top":cluster{"Top":dbl[], "Top":dbl[]}[])
      n116 = for {
        tunnel: w245 -> [w323] mode=indexing
        tunnel: [w319] -> w244 mode=indexing
        tunnel: [w318] -> w243 mode=indexing
        n117 = Index Array(array=w323, index=0) -> (element=w320:dbl)
        n118 = Index Array(array=w323, index=1) -> (element=w321:dbl)
        n119 = Subtract(x=w320, y=-258.0) -> (x-y=w327:dbl)
        n120 = Absolute Value(x=w327) -> (abs(x)=w326:dbl)
        n121 = Less?(x=w326, y=10.0) -> (x < y?=w324:bool)
        n122 = case shown="False" w324 {
          tunnel: w321 -> [_ w331]
          tunnel: w320 -> [_ w332]
          tunnel: [w330 w332] -> w319
          tunnel: [w330 w331] -> w318
          frame False {
            w330 = nan
          }
          frame True {
          }
        }
      }
      n123 = for {
        tunnel: w282 -> [w336] mode=indexing
        tunnel: [w335] -> w281 mode=indexing
        n124 = Unbundle(w336) -> (w335:dbl)  [unwired: 1 out]
      }
      "Bottom \nResiduals (um)" <- w281
      n125 = Build Array(w290, w271, w259) -> (→"Bottom":cluster{"Bottom":dbl[], "Bottom":dbl[]}[])
      n126 = for {
        tunnel: w277 -> [w334] mode=indexing
        tunnel: [w333] -> w276 mode=indexing
        n127 = Unbundle(w334) -> (w333:dbl)  [unwired: 1 out]
      }
      "Top \nResiduals (um)" <- w276
      n128 = Index Array(array=w207, index (col)=1) -> (element=w238:dbl[])  [unwired: 1 in]
      n129 = Index Array(array=w207, index (col)=0) -> (element=w240:dbl[])  [unwired: 1 in]
      n130 = Decimate 1D Array(w238) -> (w223:dbl[], w222:dbl[], w221:dbl[], w220:dbl[], w219:dbl[], w218:dbl[], w217:dbl[], w216:dbl[], w215:dbl[], w214:dbl[], w213:dbl[], w212:dbl[], w211:dbl[], w210:dbl[])
      n131 = Decimate 1D Array(w240) -> (w237:dbl[], w236:dbl[], w235:dbl[], w234:dbl[], w233:dbl[], w232:dbl[], w231:dbl[], w230:dbl[], w229:dbl[], w228:dbl[], w227:dbl[], w226:dbl[], w225:dbl[], w224:dbl[])
      n132 = Index Array(array=w312, index #1=0, index #2=1, index #3=2, index #4=3, index #5=4, index #6=5) -> (element #1=w311:errorcluster, element #2=w310:errorcluster, element #3=w309:errorcluster, element #4=w308:errorcluster, element #5=w307:errorcluster, element #6=w306:errorcluster)
      n133 = Multiply(x=w247, y=1000.0) -> (x*y=→"Top Slope\n(um/mm)":dbl)
      n134 = Multiply(x=w250, y=1000.0) -> (x*y=→"Bottom Slope\n(um/mm)":dbl)
      n135 = Merge Errors(w311, w310, w309, w308, w307, w306) -> (w313:errorcluster)
      n136 = Bundle(w208, w210) -> (→"Fiducial 14 X":cluster{i32[], dbl[]})  [unwired: 1 in]
      n137 = Bundle(w208, w223) -> (→"Fiducial 1 X":cluster{i32[], dbl[]})  [unwired: 1 in]
      n138 = Bundle(w208, w222) -> (→"Fiducial 2 X":cluster{i32[], dbl[]})  [unwired: 1 in]
      n139 = Bundle(w208, w221) -> (→"Fiducial 3 X":cluster{i32[], dbl[]})  [unwired: 1 in]
      n140 = Bundle(w208, w220) -> (→"Fiducial 4 X":cluster{i32[], dbl[]})  [unwired: 1 in]
      n141 = Bundle(w208, w219) -> (→"Fiducial 5 X":cluster{i32[], dbl[]})  [unwired: 1 in]
      n142 = Bundle(w208, w218) -> (→"Fiducial 6 X":cluster{i32[], dbl[]})  [unwired: 1 in]
      n143 = Bundle(w208, w217) -> (→"Fiducial 7 X":cluster{i32[], dbl[]})  [unwired: 1 in]
      n144 = Bundle(w208, w216) -> (→"Fiducial 8 X":cluster{i32[], dbl[]})  [unwired: 1 in]
      n145 = Bundle(w208, w215) -> (→"Fiducial 9 X":cluster{i32[], dbl[]})  [unwired: 1 in]
      n146 = Bundle(w208, w214) -> (→"Fiducial 10 X":cluster{i32[], dbl[]})  [unwired: 1 in]
      n147 = Bundle(w208, w213) -> (→"Fiducial 11 X":cluster{i32[], dbl[]})  [unwired: 1 in]
      n148 = Bundle(w208, w212) -> (→"Fiducial 12 X":cluster{i32[], dbl[]})  [unwired: 1 in]
      n149 = Bundle(w208, w211) -> (→"Fiducial 13 X":cluster{i32[], dbl[]})  [unwired: 1 in]
      n150 = Bundle(w208, w237) -> (→"Fiducial 1 Y":cluster{i32[], dbl[]})  [unwired: 1 in]
      n151 = Bundle(w208, w236) -> (→"Fiducial 2 Y":cluster{i32[], dbl[]})  [unwired: 1 in]
      n152 = Bundle(w208, w235) -> (→"Fiducial 3 Y":cluster{i32[], dbl[]})  [unwired: 1 in]
      n153 = Bundle(w208, w234) -> (→"Fiducial 4 Y":cluster{i32[], dbl[]})  [unwired: 1 in]
      n154 = Bundle(w208, w233) -> (→"Fiducial 5 Y":cluster{i32[], dbl[]})  [unwired: 1 in]
      n155 = Bundle(w208, w232) -> (→"Fiducial 6 Y":cluster{i32[], dbl[]})  [unwired: 1 in]
      n156 = Bundle(w208, w231) -> (→"Fiducial 7 Y":cluster{i32[], dbl[]})  [unwired: 1 in]
      n157 = Bundle(w208, w230) -> (→"Fiducial 8 Y":cluster{i32[], dbl[]})  [unwired: 1 in]
      n158 = Bundle(w208, w229) -> (→"Fiducial 9 Y":cluster{i32[], dbl[]})  [unwired: 1 in]
      n159 = Bundle(w208, w228) -> (→"Fiducial 10 Y":cluster{i32[], dbl[]})  [unwired: 1 in]
      n160 = Bundle(w208, w227) -> (→"Fiducial 11 Y":cluster{i32[], dbl[]})  [unwired: 1 in]
      n161 = Bundle(w208, w226) -> (→"Fiducial 12 Y":cluster{i32[], dbl[]})  [unwired: 1 in]
      n162 = Bundle(w208, w225) -> (→"Fiducial 13 Y":cluster{i32[], dbl[]})  [unwired: 1 in]
      n163 = Bundle(w208, w224) -> (→"Fiducial 14 Y":cluster{i32[], dbl[]})  [unwired: 1 in]
      n164 = Bundle(w244, w243) -> (→"Drift 2":cluster{dbl[], dbl[]})  [unwired: 1 in]
    }
    frame #2 {
      # "CLEAN UP"
      n165 = flat-sequence {
        frame #0 {
          n166 = local read "Fiducial Loc"() -> (w380:dbl[][])
          n167 = Index Array(array=w380, index (col)=0) -> (element=w377:dbl[])  [unwired: 1 in]
          n168 = Index Array(array=w380, index (col)=1) -> (element=w378:dbl[])  [unwired: 1 in]
          n169 = Decimate 1D Array(w377) -> (w376:dbl[], w375:dbl[], w374:dbl[], w373:dbl[], w372:dbl[], w371:dbl[], w370:dbl[], w369:dbl[], w368:dbl[], w367:dbl[], w366:dbl[], w365:dbl[], w364:dbl[], w363:dbl[])
          n170 = Decimate 1D Array(w378) -> (w362:dbl[], w361:dbl[], w360:dbl[], w359:dbl[], w358:dbl[], w357:dbl[], w356:dbl[], w355:dbl[], w354:dbl[], w353:dbl[], w352:dbl[], w351:dbl[], w350:dbl[], w349:dbl[])
          n171 = Build Array(w376, w375, w374, w373, w372, w371, w370, w369, w368, w367, w366, w365, w364, w363) -> (w348:dbl[][])
          n172 = Build Array(w362, w361, w360, w359, w358, w357, w356, w355, w354, w353, w352, w351, w350, w349) -> (w347:dbl[][])
          n173 = for {
            tunnel: w348 -> [w389] mode=indexing
            tunnel: w347 -> [w388] mode=indexing
            tunnel: [w385] -> w346 mode=indexing
            tunnel: [w382] -> w345 mode=indexing
            n174 = call <vilib>:"Std Deviation and Variance.vi"("X"=w389) -> ("mean"=w387:dbl, "standard deviation"=w384:dbl)  [unwired: 1 in, 1 out]
            n175 = call <vilib>:"Std Deviation and Variance.vi"("X"=w388) -> ("mean"=w386:dbl, "standard deviation"=w383:dbl)  [unwired: 1 in, 1 out]
            n176 = Build Array(w387, w386) -> (w385:dbl[])
            n177 = Build Array(w384, w383) -> (w382:dbl[])
          }
          "Mean Location (mm)" <- w346
          n178 = Multiply(x=w345, y=1000.0) -> (x*y=→"Mean Location Error (um)":dbl[][])
        }
        frame #1 {
          n179 = local read "Mean Location (mm)"() -> (w391:dbl[][])
          n180 = for {
            tunnel: w391 -> [w406] mode=indexing
            tunnel: [w392] -> w390 mode=indexing
            n181 = Index Array(array=w406, index #1=0, index #2=1) -> (element #1=w399:dbl, element #2=w396:dbl)
            n182 = Greater?(x=w396, y=-90.0) -> (0:w405:bool)
            n183 = case shown="True" w405 {
              tunnel: [w409 w411] -> w402
              tunnel: [w408 w410] -> w398
              frame False {
                n184 = local read "Top Slope\n(um/mm)"() -> (w409:dbl)
                n185 = local read "Top Intercept\n(mm)"() -> (w408:dbl)
              }
              frame True {
                n186 = local read "Bottom Intercept\n(mm)"() -> (w410:dbl)
                n187 = local read "Bottom Slope\n(um/mm)"() -> (w411:dbl)
              }
            }
            n188 = Divide(x=w402, y=1000.0) -> (x/y=w400:dbl)
            n189 = Multiply(x=w399, y=w400) -> (x*y=w397:dbl)
            n190 = Add(x=w397, y=w398) -> (x+y=w395:dbl)
            n191 = Subtract(x=w396, y=w395) -> (x-y=w394:dbl)
            n192 = Multiply(x=w394, y=1000.0) -> (x*y=w392:dbl)
          }
          "Deviation from Fit (um)" <- w390
        }
        frame #2 {
          n193 = local read "Deviation from Fit (um)"() -> (w414:dbl[])
          n194 = for {
            N: 6 -> [_]
            tunnel: [w426] -> w419 mode=indexing
            i -> [w423]
            n195 = local read "Mean Location (mm)"() -> (w439:dbl[][])
            n196 = Add(x=7, y=w423) -> (x+y=w425:i32)
            n197 = Add(x=w425, y=1) -> (x+y=w438:i32)
            n198 = Index Array(array=w439, index (row)=w425) -> (element=w436:dbl[])  [unwired: 1 in]
            n199 = Index Array(array=w439, index (row)=w438) -> (element=w435:dbl[])  [unwired: 1 in]
            n200 = Subtract(x=w436, y=w435) -> (x-y=w434:dbl[])
            n201 = Index Array(array=w434, index #1=0, index #2=1) -> (element #1=w431:dbl, element #2=w430:dbl)
            n202 = Square(x=w431) -> (x^2=w429:dbl)
            n203 = Square(x=w430) -> (x^2=w428:dbl)
            n204 = Add(x=w429, y=w428) -> (x+y=w427:dbl)
            n205 = Square Root(x=w427) -> (sqrt(x)=w426:dbl)
          }
          "Fiducial spacing (mm)\n(top)" <- w419
          n206 = for {
            N: 6 -> [_]
            tunnel: [w440] -> w421 mode=indexing
            i -> [w452]
            n207 = local read "Mean Location (mm)"() -> (w454:dbl[][])
            n208 = Add(x=w452, y=1) -> (x+y=w453:i32)
            n209 = Index Array(array=w454, index (row)=w452) -> (element=w450:dbl[])  [unwired: 1 in]
            n210 = Index Array(array=w454, index (row)=w453) -> (element=w449:dbl[])  [unwired: 1 in]
            n211 = Subtract(x=w450, y=w449) -> (x-y=w448:dbl[])
            n212 = Index Array(array=w448, index #1=0, index #2=1) -> (element #1=w445:dbl, element #2=w444:dbl)
            n213 = Square(x=w445) -> (x^2=w443:dbl)
            n214 = Square(x=w444) -> (x^2=w442:dbl)
            n215 = Add(x=w443, y=w442) -> (x+y=w441:dbl)
            n216 = Square Root(x=w441) -> (sqrt(x)=w440:dbl)
          }
          "Fiducial spacing (mm)\n(bottom)" <- w421
          n217 = call <vilib>:"General Histogram.vi"("X"=w414, "max"=75.0, "min"=-75.0, "# bins"=10) -> ("Histogram Graph"=→"Fit Deviation":T1)  [unwired: 7 in, 4 out]
          n218 = call <vilib>:"Std Deviation and Variance.vi"("X"=w414) -> ("mean"=→"Mean":dbl, "standard deviation"=→"Std Dev":dbl)  [unwired: 1 in, 1 out]
        }
      }
      n219 = event shown="[1] \"Stop and delete\": Value Change" {
        selector: _ -> [_ _]
        dyn-events: _ -> [_ _]
        timeout: _ -> [_ _]
        tunnel: [_ w460] -> w340
        tunnel: w339 -> [_ w457]
        tunnel: [_ w456] -> w338
        tunnel: w337 -> [_ w455]
        event Timeout {
          n220 = event-data() -> ()  [unwired: 1 in, 2 out]
        }
        event "Stop and delete": Value Change {
          n221 = event-data() -> ()  [unwired: 1 in, 2 out]
          n222 = flat-sequence {
            tunnel: [w467] -> w459
            tunnel: [w466] -> w458
            tunnel: w457 -> [w465]
            tunnel: w455 -> [w461]
            tunnel: [w462] -> w456
            tunnel: [w470] -> w460
            tunnel: w459 -> [w470]
            tunnel: w458 -> [w469]
            frame #0 {
              w466 = FALSE ("Review")
              n223 = local read "Template Image"() -> (w468:T4)
              n224 = local read "Selected subarray"() -> (w464:T4)
              n225 = call "DumpImageSet (SubVI).vi"("error in (no error)"=w461, "Calibrated Image Array"=w465) -> ("error out"=w463:errorcluster)  [unwired: 6 in]
              n226 = local write "Review"(w466) -> ()
              n227 = call "IMAQ Dispose"("Image"=w468, "error in (no error)"=w463) -> ("error out"=w467:errorcluster)  [unwired: 4 in]
              n228 = call "IMAQ Dispose"("Image"=w464, "error in (no error)"=w463) -> ("error out"=w462:errorcluster)  [unwired: 4 in]
            }
            frame #1 {
              n229 = local write "Stop and delete"(w469) -> ()
            }
          }
        }
      }
      n230 = local write "Search running?"(FALSE ("Search running?")) -> ()
      "Review" <- TRUE ("Review")
    }
  }
  n231 = Merge Errors(w18, w10) -> (w17:errorcluster)
  n232 = call <vilib>:"General Error Handler.vi"("error in (no error)"=w17) -> ("error out"=→"error out":errorcluster)  [unwired: 10 in, 4 out]
